vi "Test IMAQ.vi"() -> (0 "error out":errorcluster)   [LabVIEW 2020]
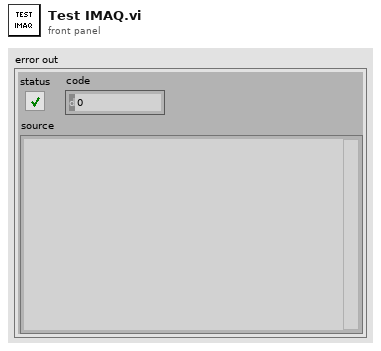
[diagram p1: front panel]
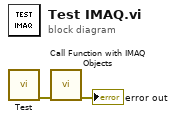
[diagram p0: block diagram]
diagram:
  n1 = call "Test.vi"() -> ("error out"=w2:errorcluster)  [unwired: 11 in]
  n2 = call "Call Function with IMAQ Objects.vi"("error in (no error)"=w2) -> ("error out"=→"error out":errorcluster)  [unwired: 10 in]
